vi "TDC_getSingleStopPreselection.vi"(8 "Error In":errorcluster) -> (0 "Error Out":errorcluster, 2 "Single Stop":bool)   [LabVIEW 2011]
uses:
  tdcbase.dll
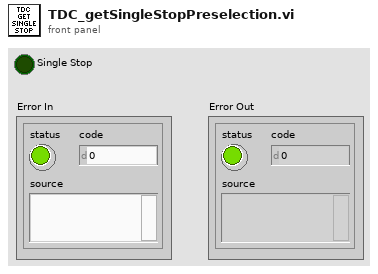
[diagram p1: front panel]
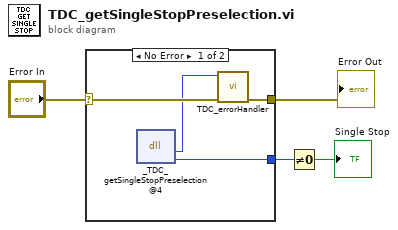
[diagram p0: block diagram]
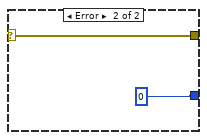
[diagram p2: hidden frame]
diagram:
  n1 = case shown="No Error" "Error In" {
    selector: "Error In" -> [w7 w10]
    tunnel: [w6 w10] -> w3
    tunnel: [w8 0] -> w2
    frame No Error {
      n2 = dll-call lib="X:/tdcbase.dll" fn="_TDC_getSingleStopPreselection@4"() -> ("return type"=w5:i32, "on"=w8:i32)  [unwired: 4 in, 2 out]
      n3 = call "TDC_errorHandler.vi"("Error In"=w7, "TDC Return Code"=w5) -> ("Error Out"=w6:errorcluster)  [unwired: 9 in]
    }
    frame Error {
    }
  }
  "Error Out" <- w3
  n4 = Not Equal To 0?(x=w2) -> (x != 0?=→"Single Stop":bool)
